vi "DetectRemotePanelConnection.vi"(4 "error in (no error)":errorcluster) -> (0 "error out":errorcluster, 2 "new connection?":bool)   [LabVIEW 2015]
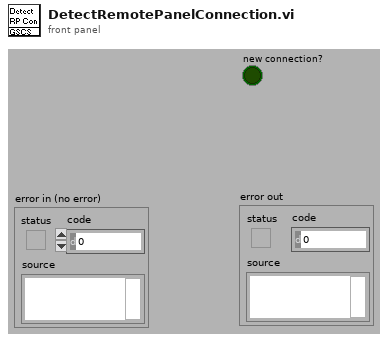
[diagram p1: front panel]
types:
  T1 = typedef "LVRemotePanelConnectionsTypeDef.ctl" = cluster{"VI Name":string, "Remote":string, "UserName":string, "Port":i32, "Status":enum32{"Viewing", "Waiting For Control", "Controlling"}, "Create Time":timestamp, "Status Time":timestamp, "Control End Time":timestamp}[]
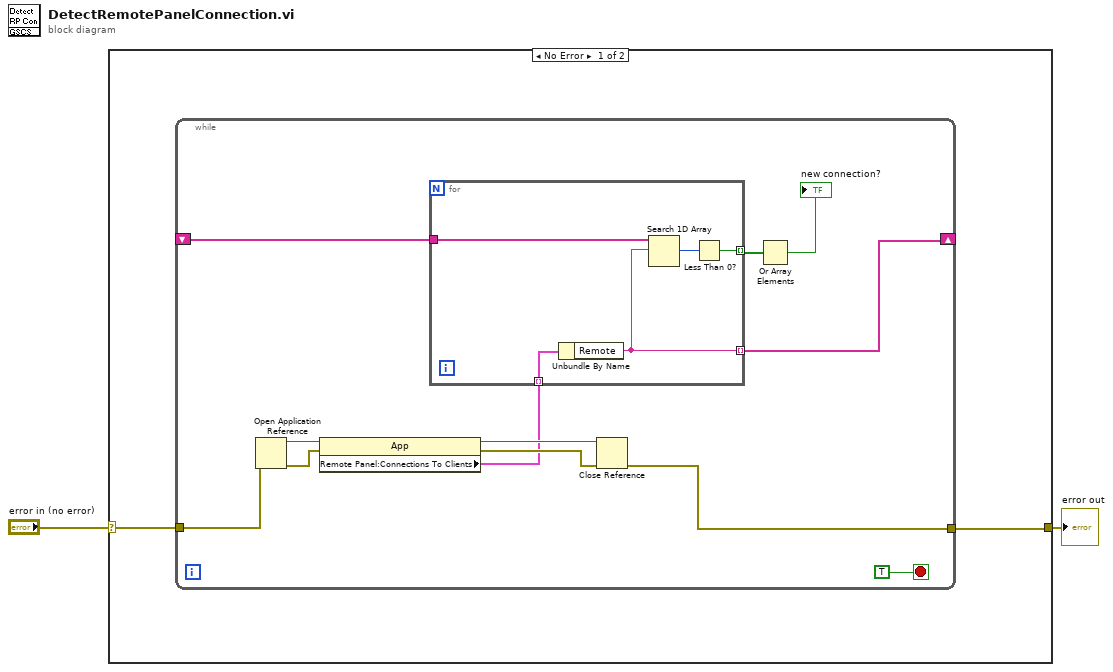
[diagram p0: block diagram]
diagram:
  n1 = case shown="No Error" "error in (no error)" {
    selector: "error in (no error)" -> [w4 w22]
    tunnel: [w3 w22] -> w1
    frame No Error {
      n2 = while {
        tunnel: w4 -> [w16]
        shift-right: [w8] -> _
        shift-left: _ -> [w7]
        tunnel: [w10] -> w3
        stop <- TRUE stop-if-true
        n3 = Open Application Reference(8:w16) -> (0:w14:errorcluster, 3:w15:refnum<vi>)  [unwired: 3 in]
        n4 = property class="App"(reference=w15, error in=w14) -> (reference out=w12:refnum<vi>, error out=w11:errorcluster, "Remote Panel:Connections To Clients"=w9:T1)
        n5 = for {
          tunnel: w9 -> [w21] mode=indexing
          tunnel: [w19] -> w8 mode=indexing
          tunnel: w7 -> [w20]
          tunnel: [w17] -> w6 mode=indexing
          n6 = Unbundle By Name(w21) -> ("Remote"=w19:string)
          n7 = Search 1D Array(1D array=w20, element=w19) -> (index of element=w18:i32)  [unwired: 1 in]
          n8 = Less Than 0?(x=w18) -> (x < 0?=w17:bool)
        }
        n9 = Close Reference(reference=w12, error in (no error)=w11) -> (error out=w10:errorcluster)
        n10 = Or Array Elements(Boolean array=w6) -> (logical OR=→"new connection?":bool)
      }
    }
    frame Error {
    }
  }
  "error out" <- w1
